vi "Consecutive.vi"(9 "Boolean":bool, 10 "rms value":dbl, 11 "rms value 2":dbl) -> (1 "Array Size 3":u32, 2 "Delayed RMS2>RMS1 for 3 data":dynamicdata(graph), 3 "RMS2>RMS1 for 3 data":dynamicdata(graph))   [LabVIEW 2021]
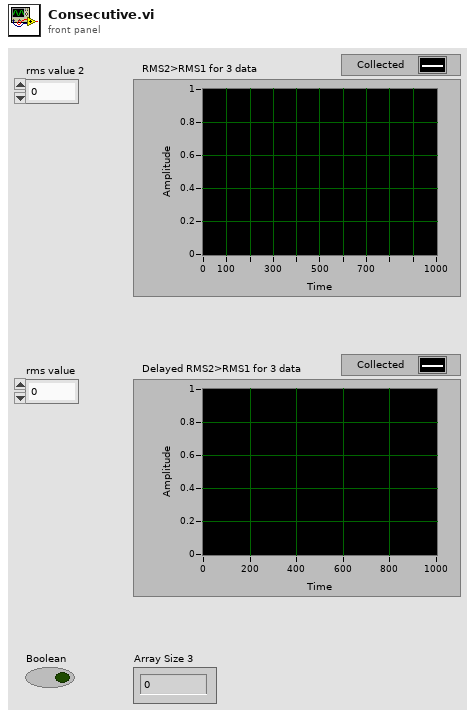
[diagram p1: front panel]
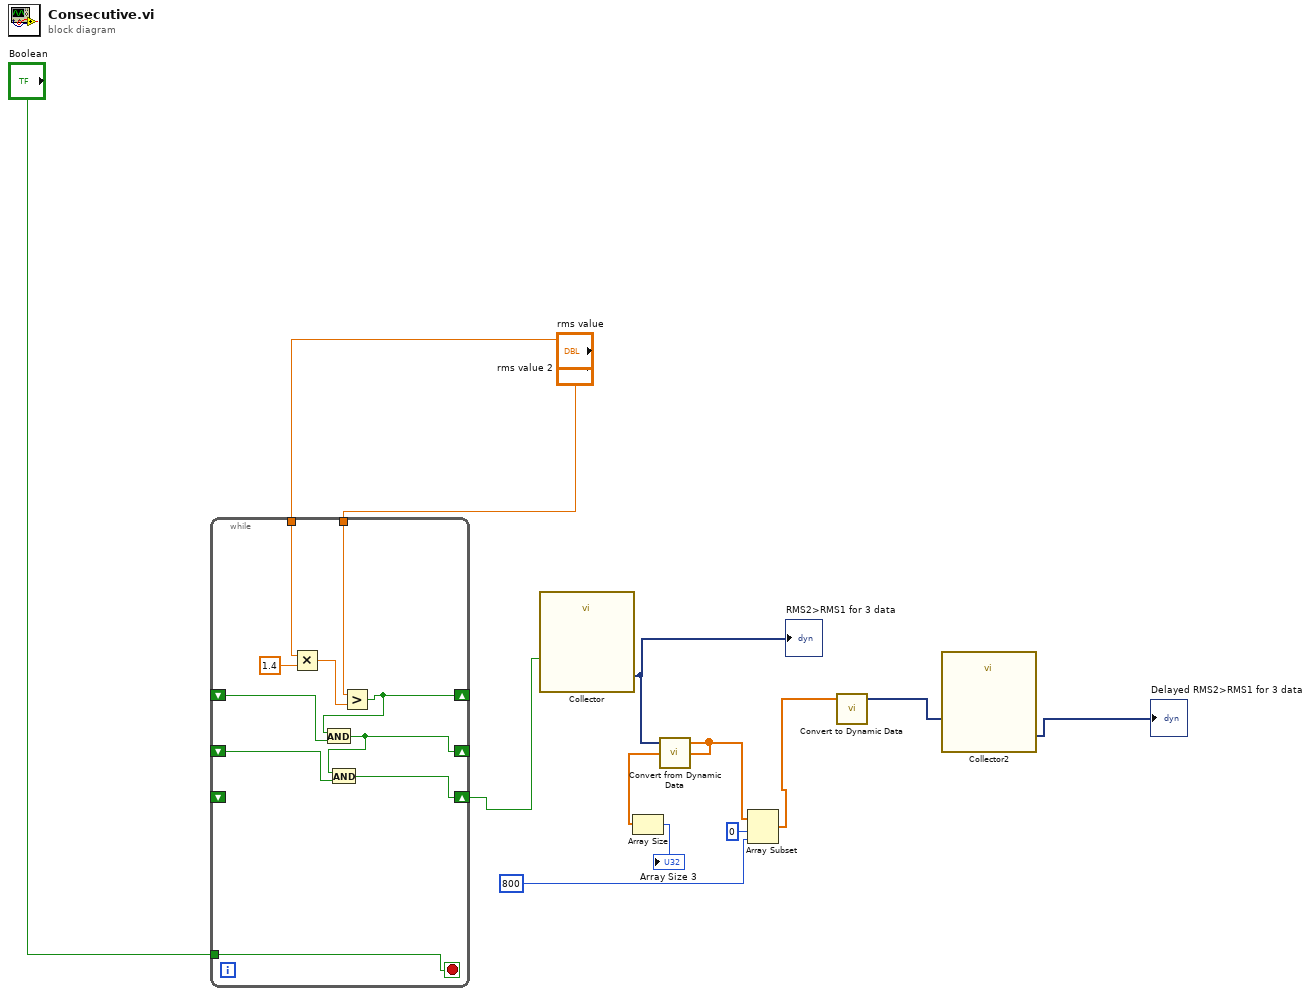
[diagram p0: block diagram]
diagram:
  n1 = while {
    tunnel: "rms value 2" -> [w20]
    tunnel: "rms value" -> [w19]
    shift-right: [w14] -> _
    shift-left: _ -> [w15]
    shift-right: [w17] -> _
    shift-left: _ -> [w16]
    tunnel: "Boolean" -> [w18]
    shift-right: [w13] -> w5
    shift-left: _ -> [_]
    stop <- w18 stop-if-true
    n2 = Multiply(x=w19, y=1.4) -> (x*y=w21:dbl)
    n3 = Greater?(x=w20, y=w21) -> (0:w17:bool)
    n4 = And(x=w17, y=w16) -> (x .and. y?=w14:bool)
    n5 = And(x=w14, y=w15) -> (x .and. y?=w13:bool)
  }
  n6 = call "Collector"("Signals"=w5) -> ("Collected Signals"=w7:dynamicdata)  [unwired: 9 in, 1 out]
  "RMS2>RMS1 for 3 data" <- w7
  n7 = call "Convert from Dynamic Data"("Dynamic Data Type"=w7) -> ("Array"=w10:dbl[])  [unwired: 3 in]
  n8 = Array Size(array=w10) -> (size(s)=→"Array Size 3":i32)
  n9 = Array Subset(array=w10, index=0, length=800 ("index")) -> (w12:dbl[])
  n10 = call "Convert to Dynamic Data"("Array"=w12) -> ("Dynamic Data Type"=w6:dynamicdata)  [unwired: 3 in]
  n11 = call "Collector2"("Signals"=w6) -> ("Collected Signals"=→"Delayed RMS2>RMS1 for 3 data":dynamicdata)  [unwired: 9 in, 1 out]
